vi "LVSCharWrt.vi"(8 "String In":string, 11 "COM Port":refnum<visa-resource-name>) -> (0 "ComError":bool)   [LabVIEW 2017]
uses:
  <vilib>/Utility/error.llb/DialogType.ctl
  instr.lib/lvserial/lvserial.lvlib
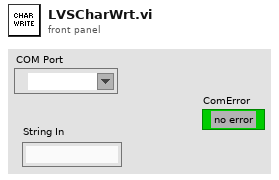
[diagram p1: front panel]
types:
  T1 = typedef "DialogType.ctl" = u16
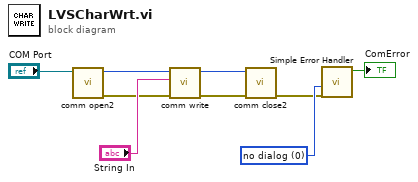
[diagram p0: block diagram]
diagram:
  w3 = T1 0 items=["no dialog", "OK message", "continue or stop message", "OK message + warnings", "continue/stop + warnings"] ("type of dialog (OK msg:1)")
  n1 = call "comm open2.vi"("Comm Port Name"="COM Port") -> ("error out"=w7:errorcluster, "Comm Handle"=w6:u32)  [unwired: 4 in, 1 out]
  n2 = call "comm write.vi"("error in (no error)"=w7, "string to write"="String In", "Comm Handle"=w6) -> ("error out"=w4:errorcluster, "dup Comm Handle"=w5:u32)  [unwired: 6 in, 1 out]
  n3 = call "comm close2.vi"("error in (no error)"=w4, "Comm Handle"=w5) -> ("error out"=w1:errorcluster)  [unwired: 5 in]
  n4 = call <vilib>:"Simple Error Handler.vi"("type of dialog (OK msg:1)"=w3, "error in (no error)"=w1) -> ("error?"=→"ComError":bool)  [unwired: 7 out]
